vi "Main.vi"() -> ()   [LabVIEW 2013]
panel:
  in  "退出系统":bool
  in  "串口助手":bool
  in  "姿态助手":bool
  in  "视觉平台":bool
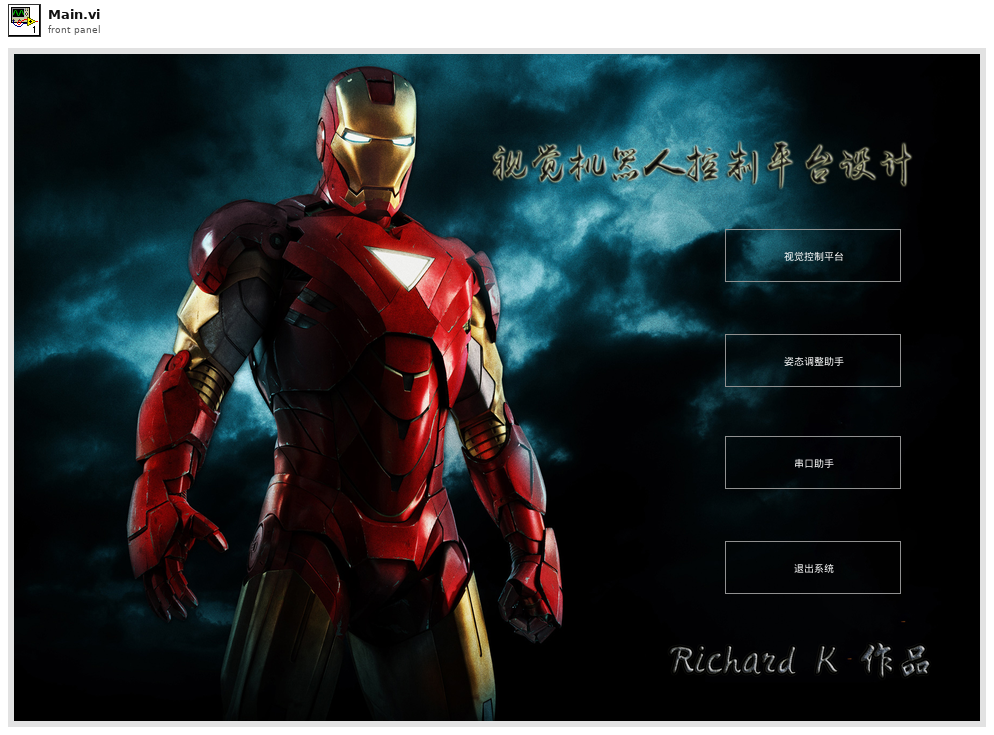
[diagram p1: front panel]
types:
  T1 = enum32{"Invalid", "Standard", "Closed", "Hidden", "Minimized", "Maximized"}
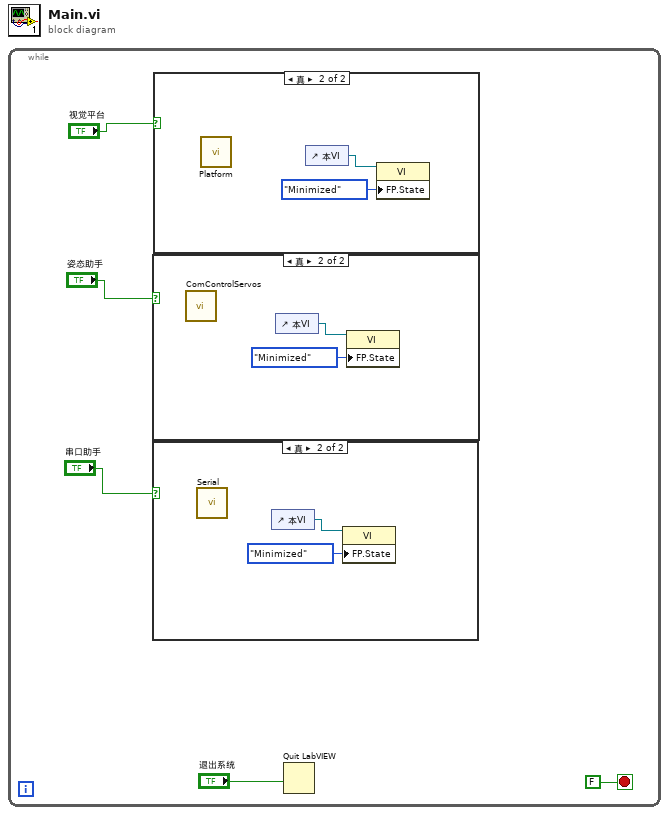
[diagram p0: block diagram]
diagram:
  n1 = while {
    stop <- FALSE stop-if-true
    n2 = case shown="真" "姿态助手" {
      frame False {
      }
      frame True {
        n3 = call "ComControlServos.vi"() -> ()  [unwired: 1 in]
        n4 = control-ref of="本VI"() -> (w8:refnum<vi>)
        n5 = property class="VI"(reference=w8, "FP.State"=T1."Minimized" ("前面板窗口:状态")) -> ()  [unwired: 1 in, 2 out]
      }
    }
    n6 = case shown="真" "串口助手" {
      frame False {
      }
      frame True {
        n7 = call "Serial.vi"() -> ()  [unwired: 12 in]
        n8 = control-ref of="本VI"() -> (w7:refnum<vi>)
        n9 = property class="VI"(reference=w7, "FP.State"=T1."Minimized" ("前面板窗口:状态")) -> ()  [unwired: 1 in, 2 out]
      }
    }
    n10 = case shown="真" "视觉平台" {
      frame False {
      }
      frame True {
        n11 = call "Platform.vi"() -> ()  [unwired: 12 in]
        n12 = control-ref of="本VI"() -> (w11:refnum<vi>)
        n13 = property class="VI"(reference=w11, "FP.State"=T1."Minimized" ("前面板窗口:状态")) -> ()  [unwired: 1 in, 2 out]
      }
    }
    n14 = Quit LabVIEW(quit? (T)="退出系统") -> ()
  }
